vi "Init from Ref.vi"(8 "error in":errorcluster, 10 "Cell":refnum<k24>, 11 "Check Box in":refnum<class "Check Box.lvclass">) -> (0 "error out":errorcluster, 3 "Check Box out":refnum<class "Check Box.lvclass">)   [LabVIEW 2023, in "SourceGrid.lvlib" / "Check Box.lvclass"]
uses:
  Check Box.lvclass
  D:/git/Sourcegrid-LabVIEW/dll/SourceGrid.dll
  dll/SourceGrid.dll
  Cell/Cell.lvclass
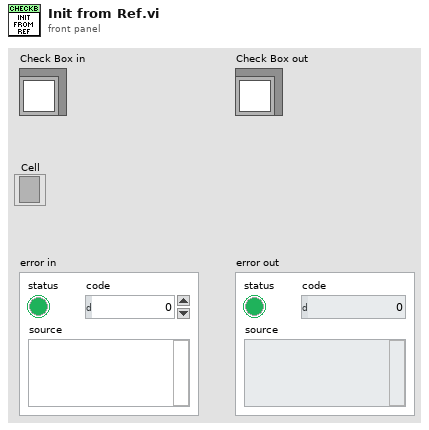
[diagram p1: front panel]
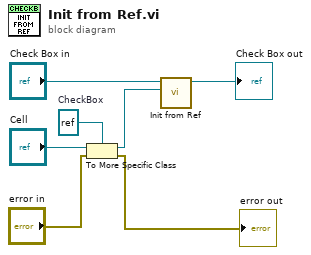
[diagram p0: block diagram]
diagram:
  w4 = refnum<k24> refnum  # CheckBox
  n1 = To More Specific Class(target class=w4, reference="Cell", error in="error in") -> (specific class reference=w2:refnum<k24>, error out=→"error out":errorcluster)
  n2 = call-parent "Init from Ref.vi"("Cell"=w2, "Cell in"="Check Box in") -> ("Cell out"=→"Check Box out":refnum<class "Check Box.lvclass">)  [unwired: 8 in, 1 out]
